vi "12_rand no using timer.vi"() -> ()   [LabVIEW 2018]
panel:
  out "Numeric Float":dbl
  # "Develop HMI (Human Machine Interface) to display random number from 0 to 99\nusing for loop for only 5 times with timer 0.5 mili sec"
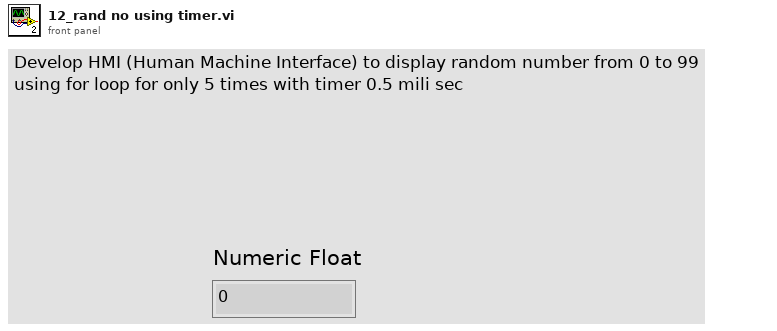
[diagram p1: front panel]
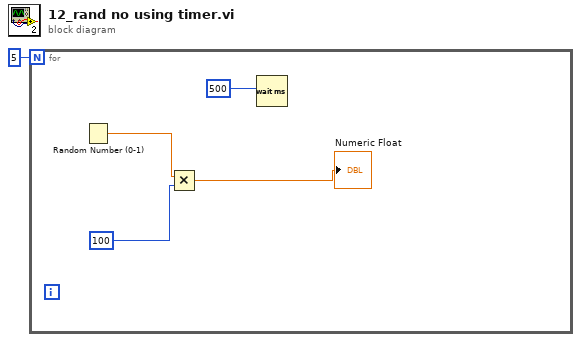
[diagram p0: block diagram]
diagram:
  n1 = for {
    N: 5 -> [_]
    n2 = Random Number (0-1)() -> (number: 0 to 1=w5:dbl)
    n3 = Multiply(x=w5, y=100) -> (x*y=→"Numeric Float":dbl)
    n4 = Wait (ms)(milliseconds to wait=u32 500 ("millisecond timer value")) -> ()  [unwired: 1 out]
  }
